vi "SDCP BTR.vi"(6 "Command":enum16{"Load", "Acquire"}(ring), 8 "error in (no error)":errorcluster, 9 "Block transfer parameters file path":path, 10 "Number of transfers":u16, 11 "Parameter IDs":u8[](array[numeric])) -> (0 "error out":errorcluster, 1 "BTRP out":T1[](array[typedef]), 2 "Status":T3, 3 "Read BTR parameters":T1[](array[typedef]))   [LabVIEW 2020]
uses:
  Typedefs/SDCP BTR Params.ctl
  Typedefs/SDCP BTR Parameter cluster.ctl
  Typedefs/SDCP BTR Parameter data type.ctl
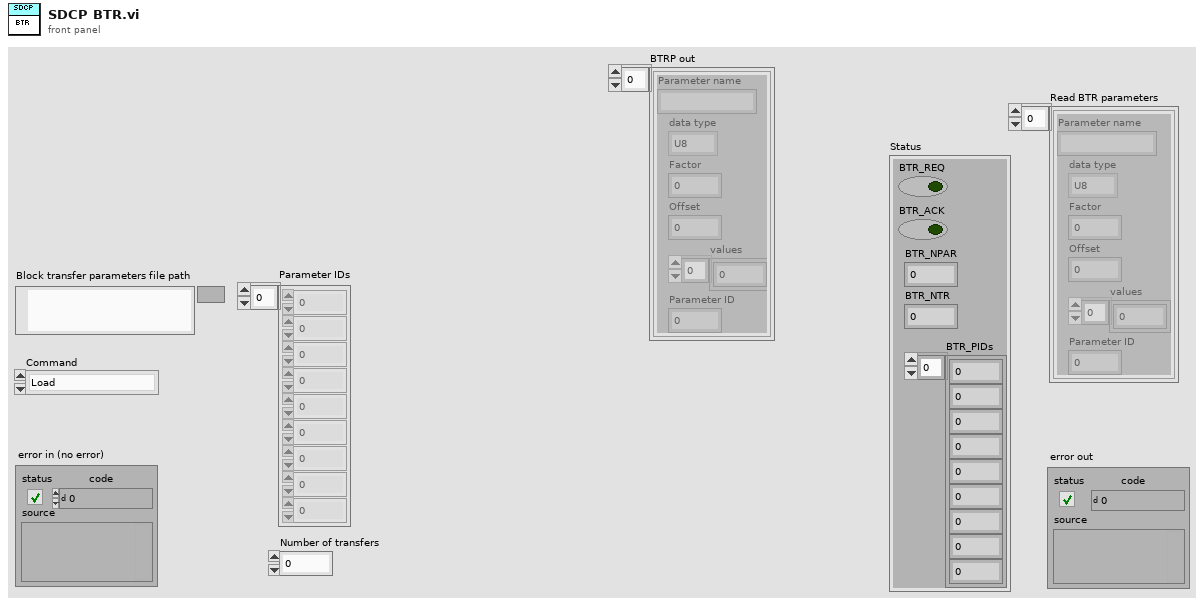
[diagram p1: front panel]
types:
  T1 = typedef "SDCP BTR Parameter cluster.ctl" = cluster{"Parameter name":string, "data type":T2, "Factor":dbl, "Offset":dbl, "values":dbl[], "Parameter ID":i32}
  T2 = typedef "SDCP BTR Parameter data type.ctl" = enum16{"U8", "I8", "U16", "I16", "U32", "I32", "F32"}
  T3 = typedef "SDCP BTR Params.ctl" = cluster{"BTR_REQ":bool, "BTR_ACK":bool, "BTR_NPAR":i32, "BTR_NTR":i32, "BTR_PIDs":u8[]}
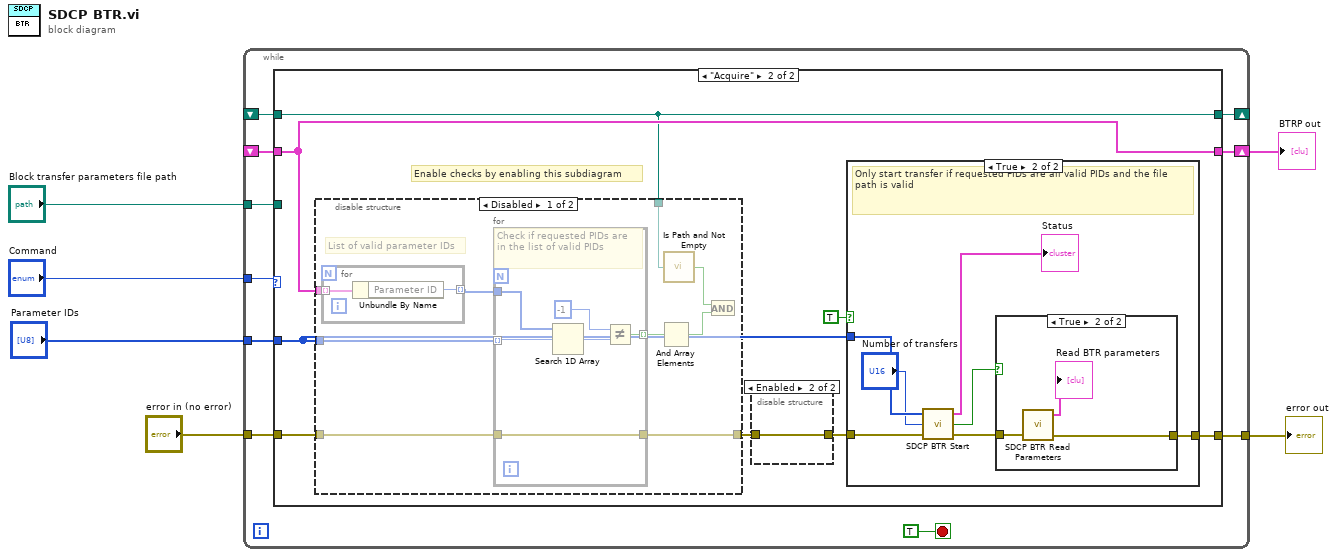
[diagram p0: block diagram]
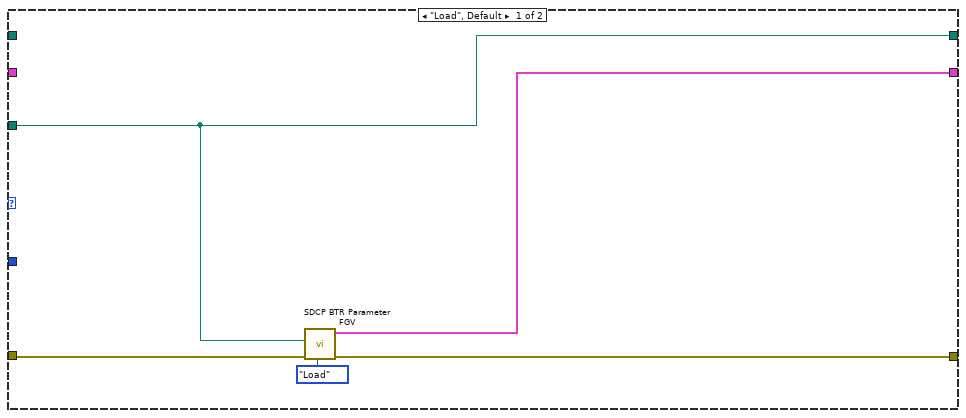
[diagram p2: hidden frame]
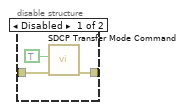
[diagram p3: hidden frame]
diagram:
  n1 = while {
    tunnel: "error in (no error)" -> [w14]
    shift-right: [w12] -> _
    shift-left: _ -> [w10]
    tunnel: "Command" -> [w15]
    tunnel: "Block transfer parameters file path" -> [w13]
    tunnel: [w11] -> w3
    tunnel: "Parameter IDs" -> [w9]
    shift-right: [w8] -> w1
    shift-left: _ -> [w7]
    stop <- TRUE stop-if-true
    n2 = case shown="\"Acquire\"" w15 {
      tunnel: w14 -> [w21 w29]
      tunnel: w13 -> [w19 _]
      tunnel: [w19 w26] -> w12
      tunnel: [w18 w27] -> w11
      tunnel: w10 -> [_ w26]
      tunnel: w9 -> [_ w24]
      tunnel: [w17 w28] -> w8
      tunnel: w7 -> [_ w28]
      frame "Load", Default {
        n3 = call "SDCP BTR Parameter FGV.vi"("error in (no error)"=w21, "Command"=enum16{"Load", "Read", "Write"}."Load", "BTR Parameter File Path"=w19) -> ("error out"=w18:errorcluster, "BTRP out"=w17:T1[])  [unwired: 3 in]
      }
      frame "Acquire" {
        # "Enable checks by enabling this subdiagram"
        n4 = disable-structure shown="Disabled" {
          disable-tunnel: w29 -> [w42 w51]
          disable-tunnel: w28 -> [w40 _]
          disable-tunnel: [w36 w51] -> w23
          disable-tunnel: w24 -> [w35 _]
          disable-tunnel: w26 -> [w34 _]
          frame Disabled {
            # "List of valid parameter IDs"
            n5 = for {
              tunnel: w40 -> [w50] mode=indexing
              tunnel: [w49] -> w41 mode=indexing
              n6 = Unbundle By Name(w50) -> ("Parameter ID"=w49:i32)
            }
            n7 = for {
              tunnel: w42 -> [w43]
              tunnel: w35 -> [w48] mode=indexing
              tunnel: w41 -> [w47]
              tunnel: [w44] -> w39 mode=indexing
              tunnel: [w43] -> w36
              # "Check if requested PIDs are\nin the list of valid PIDs"
              n8 = Search 1D Array(1D array=w47, element=w48) -> (index of element=w46:i32)  [unwired: 1 in]
              n9 = Not Equal?(x=-1, y=w46) -> (x != y?=w44:bool)
            }
            n10 = And Array Elements(Boolean array=w39) -> (logical AND=w38:bool)
            n11 = call <vilib>:"Is Path and Not Empty.vi"("path"=w34) -> ("Is Path and Not Empty?"=w37:bool)  [unwired: 4 in]
            n12 = And(x=w37, y=w38) -> ()  [unwired: 1 out]
          }
          frame Enabled {
          }
        }
        n13 = disable-structure shown="Enabled" {
          disable-tunnel: w23 -> [w32 w33]
          disable-tunnel: [w31 w33] -> w22
          frame Disabled {
            n14 = call "SDCP Transfer Mode Command.vi"("error in (no error)"=w32, "BTR"=TRUE) -> ("error out"=w31:errorcluster)  [unwired: 5 in]
          }
          frame Enabled {
          }
        }
        n15 = case shown="True" TRUE {
          tunnel: w22 -> [w52 w59]
          tunnel: w24 -> [_ w58]
          tunnel: [w52 w55] -> w27
          frame False {
          }
          frame True {
            # "Only start transfer if requested PIDs are all valid PIDs and the file path is valid"
            n16 = call "SDCP BTR Start.vi"("error in (no error)"=w59, "Number of transfers"="Number of transfers", "Parameter IDs"=w58) -> ("error out"=w56:errorcluster, "No timeout"=w53:bool, "out"=→"Status":T3)
            n17 = case shown="True" w53 {
              tunnel: w56 -> [w60 w63]
              tunnel: [w60 w61] -> w55
              frame False {
              }
              frame True {
                n18 = call "SDCP BTR Read Parameters.vi"("error in (no error)"=w63) -> ("Read BTR parameters"=→"Read BTR parameters":T1[], "error out"=w61:errorcluster)  [unwired: 1 in, 1 out]
              }
            }
          }
        }
      }
    }
  }
  "error out" <- w3
  "BTRP out" <- w1
